vi "MTMount_monitorCommand_trackTarget.vi"(8 "error in (no error)":errorcluster, 11 "command_trackTarget_Ctl":T1) -> (0 "error out":errorcluster, 2 "function return":i32, 3 "command_trackTarget_Ctl out":T1)   [LabVIEW 2018, in "SALLV_MTMount.lvlib"]
doc: "int MTMount_shm_monitorCommand_trackTargetLV(MTMount_command_trackTargetLV *command_trackTarget_Ctl );"
uses:
  SALLV_MTMount.lvlib
  DataTypes/command_trackTarget.ctl
  SALLV_MTMount.so
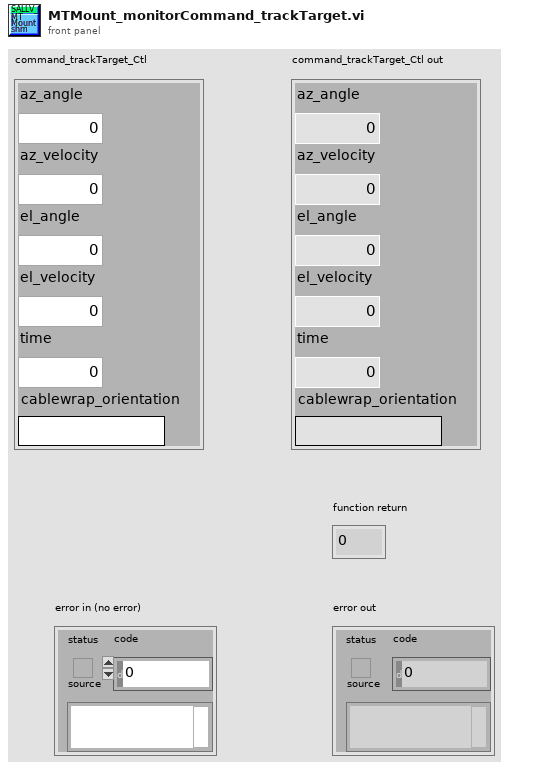
[diagram p1: front panel]
types:
  T1 = typedef "SALLV_MTMount.lvlib/command_trackTarget.ctl" = cluster{"az_angle":dbl, "az_velocity":dbl, "el_angle":dbl, "el_velocity":dbl, "time":dbl, "cablewrap_orientation":string}
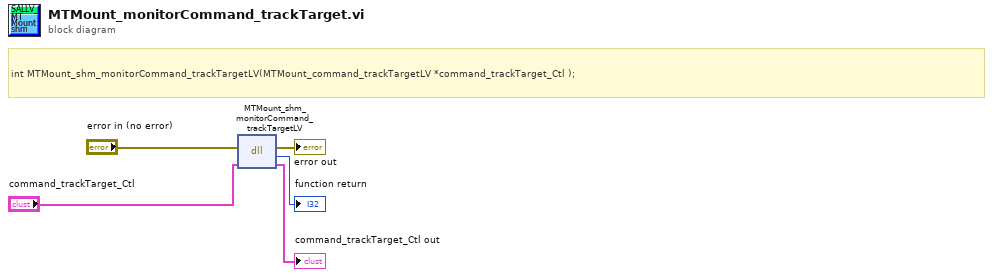
[diagram p0: block diagram]
diagram:
  # "int MTMount_shm_monitorCommand_trackTargetLV(MTMount_command_trackTargetLV *command_trackTarget_Ctl );"
  n1 = dll-call lib="home/ttsai/Document/salApiMTMount/SALLV_MTMount/SALLV_MTMount.*" fn="MTMount_shm_monitorCommand_trackTargetLV"(error in="error in (no error)", "command_trackTarget_Ctl"="command_trackTarget_Ctl") -> (error out=→"error out":errorcluster, →"function return":i32, "command_trackTarget_Ctl"=→"command_trackTarget_Ctl out":T1)  [unwired: 2 in, 1 out]
